vi "Graph Data.vi"(8 "error in (no error)":errorcluster, 10 "Graph data":dbl, 11 "Generador funciones in":refnum<class "Generador funciones.lvclass">) -> (0 "error out":errorcluster, 3 "Generador funciones out":refnum<class "Generador funciones.lvclass">)   [LabVIEW 2019, in "Generador funciones.lvlib" / "Generador funciones.lvclass"]
uses:
  Generador funciones.lvclass
  Generador funciones.lvclass/Generador funciones.ctl
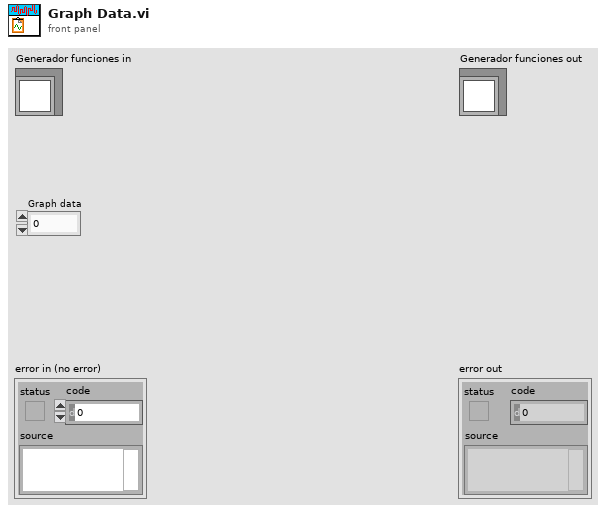
[diagram p1: front panel]
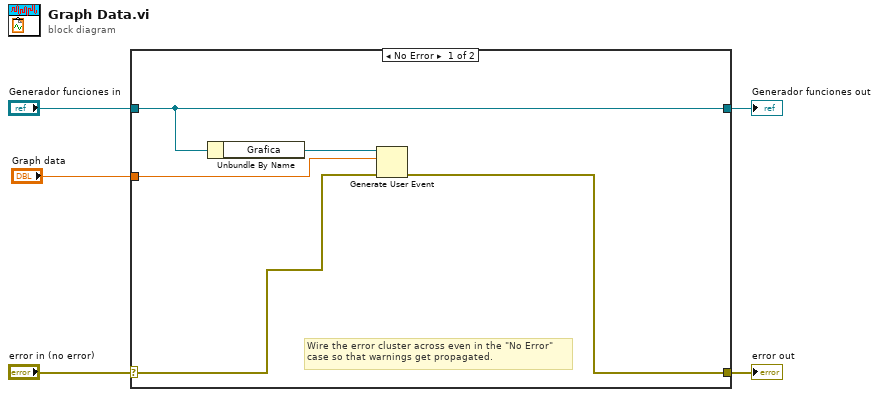
[diagram p0: block diagram]
diagram:
  n1 = case shown="No Error" "error in (no error)" {
    selector: "error in (no error)" -> [w7 w12]
    tunnel: [w6 w12] -> w4
    tunnel: [w10 w11] -> w2
    tunnel: "Generador funciones in" -> [w10 w11]
    tunnel: "Graph data" -> [w8 _]
    frame No Error {
      # "Wire the error cluster across even in the \"No Error\"\ncase so that warnings get propagated."
      n2 = Unbundle By Name(w10) -> ("Grafica"=w9:refnum<user-event>)
      n3 = Generate User Event(user event=w9, event data cluster=w8, error in=w7) -> (error out=w6:errorcluster)  [unwired: 1 in, 1 out]
    }
    frame Error {
    }
  }
  "error out" <- w4
  "Generador funciones out" <- w2
